vi "SDG60ConfArbWaveformOLD.vi"(0 "VISA resource name":refnum<visa-resource-name>="USB0::0xF4EC::0x1101::SDG6XEBC5R0119::INSTR", 1 "Freq/SR/P (1 Hz)":dbl=1000.0 min=1e-06 max=160000000.0 step=1.0 format="%#.15g", 2 "Phase (0.0 degrees)":dbl min=-360.0 max=360.0 format="%#.15g", 3 "Interpolation 0: Zero-order":i32(ring) items=["Zero-Order", "Linear", "Sinc", "Sin27", "Sinc13"], 5 "Select Channel (1:Channel 1)":i32(ring)=1 items=["Channel 1"=1, "Channel 2"=2], 7 "Amplitude (1.0 Vpp)":dbl=1.0 min=0.001 max=20.0 step=1.0 format="%#.15f", 9 "Select Freq/SR/P":i32(ring)=1 items=["Frequency", "Sample Rate", "Period"], 11 "error in (no error)":errorcluster, 12 "DC Offset (0.00 V)":dbl min=-10.0 max=10.0 format="%#_15g", 13 "DDS/TArb 0: DDS":i32(ring) items=["DDS", "TrueArb"]) -> (4 "VISA resource name out":refnum<visa-resource-name>, 15 "error out":errorcluster)   [LabVIEW 2018]
doc: "Sets the waveform parameters for an arbitrary waveform. This VI should be called after <b>Create Arbitrary Waveform.vi</b> (for user defined arbitrary waveform) and <b>Select Arbitrary Waveform.vi</b>"
panel:
  # "Sinc style interpolations use virtual keys\nVirtual keys not used for zero-hold & linear"
  # "2mVpp-20Vpp"
  # "For Period, TrueArb won't show on monitor-but will use (rounded value)\nFor SR, need to use TrueArb\nTo change interpolation method, use TrueArb\nMay take time to switch to TrueArb if WFM is large"
  # "Freq (DDS): 1uHz-50MHz \nFreq (TrueArb): 1uHz- Max depends on WFM length\nSR: 1uS/s-300MSa/s\nP: 20ns-1Ms\n10 Digit precision for F & SR\n6 Digit precision for P"
  # "TODO:  Choose Freq/period\namplitude/hi\noffset/low\nphase/delay"
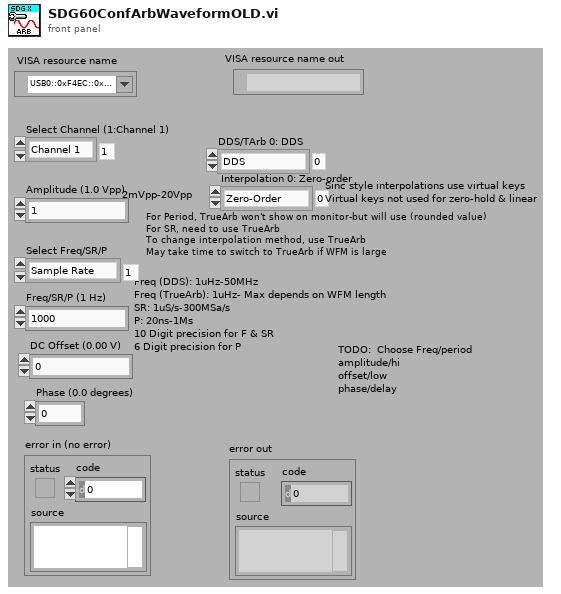
[diagram p1: front panel]
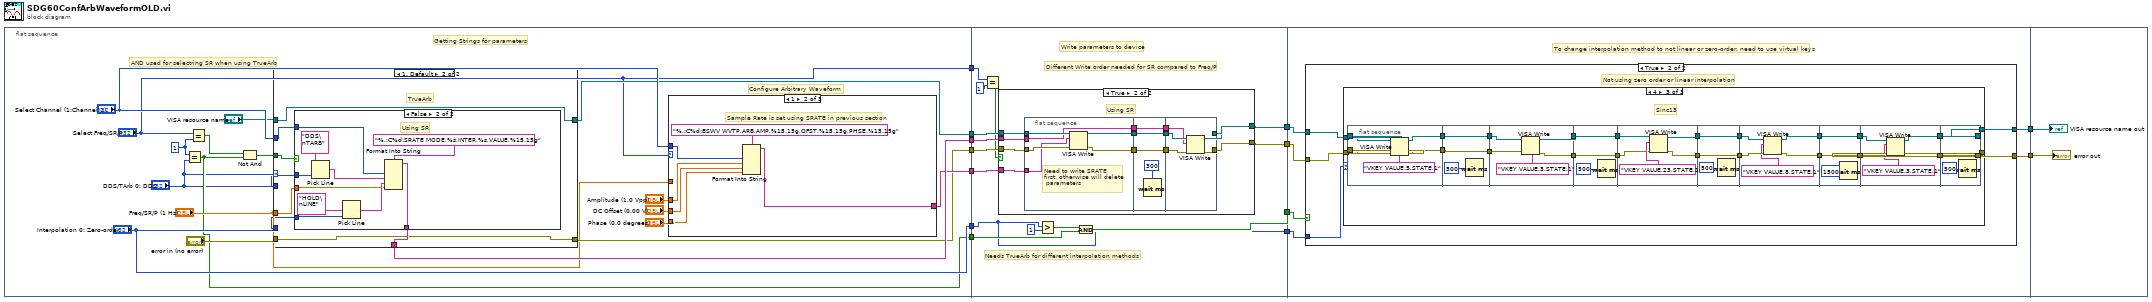
[diagram p0: block diagram]
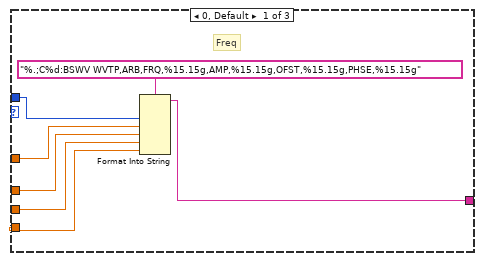
[diagram p2: hidden frame]
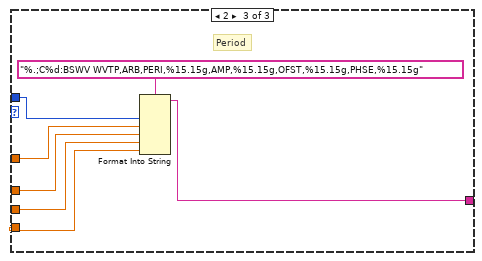
[diagram p3: hidden frame]
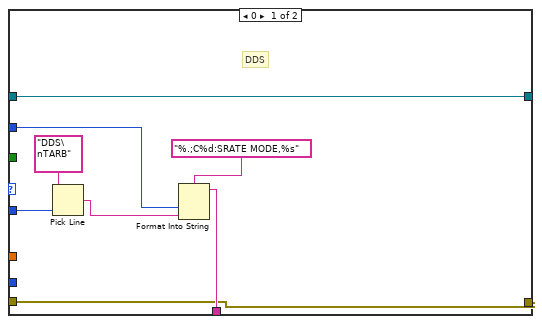
[diagram p4: hidden frame]
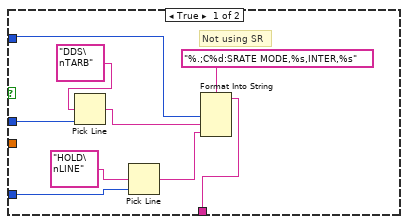
[diagram p5: hidden frame]
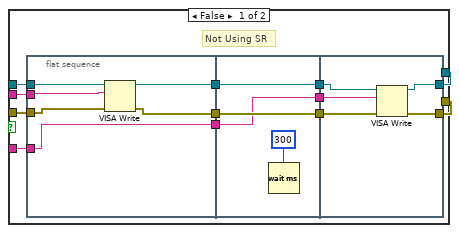
[diagram p6: hidden frame]
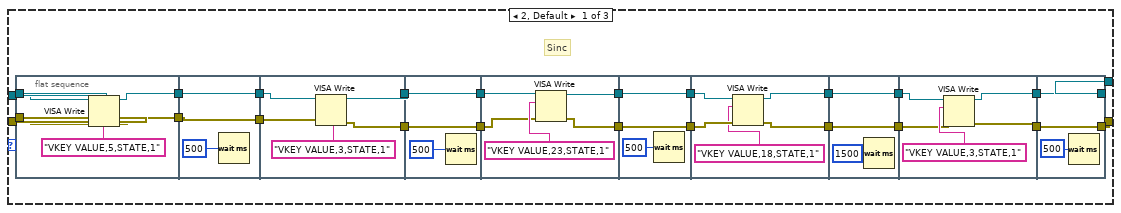
[diagram p8: hidden frame]
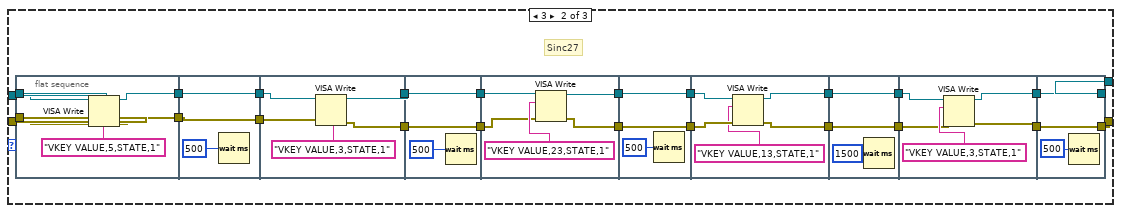
[diagram p9: hidden frame]
diagram:
  n1 = flat-sequence {
    tunnel: [w25] -> w13
    tunnel: [w24] -> w12
    tunnel: [w23] -> w11
    tunnel: [w22] -> w10
    tunnel: [w17] -> w9
    tunnel: ["Interpolation 0: Zero-order"] -> w8
    tunnel: ["Select Freq/SR/P"] -> w1
    tunnel: w13 -> [w100]
    tunnel: w12 -> [w99]
    tunnel: w11 -> [w98]
    tunnel: w10 -> [w97]
    tunnel: w9 -> [w93]
    tunnel: w8 -> [w90]
    tunnel: [w96] -> w7
    tunnel: [w95] -> w6
    tunnel: [w92] -> w5
    tunnel: [w90] -> w4
    tunnel: w1 -> [w88]
    tunnel: w7 -> [w159]
    tunnel: w6 -> [w158]
    tunnel: w5 -> [w160]
    tunnel: w4 -> [w157]
    tunnel: [w156] -> w3
    tunnel: [w155] -> w2
    tunnel: w3 -> [w354]
    tunnel: w2 -> [w355]
    frame #0 {
      w16 = 1
      # "Getting Strings for parameters"
      # "AND used for selectring SR when using TrueArb"
      # "Configure Arbitrary Waveform"
      n2 = Equal?(x=w16, y="DDS/TArb 0: DDS") -> (x = y?=w17:bool)
      n3 = Equal?(x="Select Freq/SR/P", y=w16) -> (x = y?=w18:bool)
      n4 = Not And(1:w17, 2:w18) -> (0:w15:bool)
      n5 = case shown="1, Default" "DDS/TArb 0: DDS" {
        tunnel: "Interpolation 0: Zero-order" -> [_ w67]
        tunnel: "DDS/TArb 0: DDS" -> [w58 w66]
        tunnel: "Select Channel (1:Channel 1)" -> [w56 w65]
        tunnel: [w55 w64] -> w25
        tunnel: w15 -> [_ w60]
        tunnel: "VISA resource name" -> [w53 w63]
        tunnel: "error in (no error)" -> [w52 w62]
        tunnel: [w53 w63] -> w22
        tunnel: [w52 w62] -> w23
        tunnel: "Freq/SR/P (1 Hz)" -> [_ w61]
        frame 0 {
          # "DDS"
          n6 = Pick Line(multi-line string="DDS\nTARB", line index=w58) -> (output string=w57:string)  [unwired: 1 in]
          n7 = Format Into String(format string="%.;C%d:SRATE MODE,%s", w56, w57) -> (resulting string=w55:string)  [unwired: 2 in, 1 out]
        }
        frame 1, Default {
          # "TrueArb"
          n8 = case shown="False" w60 {
            tunnel: w67 -> [w68 w85]
            tunnel: w66 -> [w70 w83]
            tunnel: w65 -> [w71 w81]
            tunnel: [w69 w80] -> w64
            tunnel: w61 -> [_ w77]
            frame True {
              # "Not using SR"
              n9 = Pick Line(multi-line string="DDS\nTARB", line index=w70) -> (output string=w76:string)  [unwired: 1 in]
              n10 = Pick Line(multi-line string="HOLD\nLINE", line index=w68) -> (output string=w75:string)  [unwired: 1 in]
              n11 = Format Into String(format string="%.;C%d:SRATE MODE,%s,INTER,%s", w71, w76, w75) -> (resulting string=w69:string)  [unwired: 2 in, 1 out]
            }
            frame False {
              # "Using SR"
              n12 = Pick Line(multi-line string="DDS\nTARB", line index=w83) -> (output string=w82:string)  [unwired: 1 in]
              n13 = Pick Line(multi-line string="HOLD\nLINE", line index=w85) -> (output string=w84:string)  [unwired: 1 in]
              n14 = Format Into String(format string="%.;C%d:SRATE MODE,%s,INTER,%s,VALUE,%15.15g", w81, w82, w84, w77) -> (resulting string=w80:string)  [unwired: 2 in, 1 out]
            }
          }
        }
      }
      n15 = case shown="1" "Select Freq/SR/P" {
        tunnel: "Freq/SR/P (1 Hz)" -> [w37 _ w50]
        tunnel: "Amplitude (1.0 Vpp)" -> [w36 w41 w49]
        tunnel: "DC Offset (0.00 V)" -> [w35 w40 w48]
        tunnel: "Phase (0.0 degrees)" -> [w34 w39 w47]
        tunnel: "Select Channel (1:Channel 1)" -> [w33 w43 w46]
        tunnel: [w32 w42 w45] -> w24
        frame 0, Default {
          # "Freq"
          n16 = Format Into String(format string="%.;C%d:BSWV WVTP,ARB,FRQ,%15.15g,AMP,%15.15g,OFST,%15.15g,PHSE,%15.15g", w33, w37, w36, w35, w34) -> (resulting string=w32:string)  [unwired: 2 in, 1 out]
        }
        frame 1 {
          # "Sample Rate is set using SRATE in previous section"
          n17 = Format Into String(format string="%.;C%d:BSWV WVTP,ARB,AMP,%15.15g,OFST,%15.15g,PHSE,%15.15g", w43, w41, w40, w39) -> (resulting string=w42:string)  [unwired: 2 in, 1 out]
        }
        frame 2 {
          # "Period"
          n18 = Format Into String(format string="%.;C%d:BSWV WVTP,ARB,PERI,%15.15g,AMP,%15.15g,OFST,%15.15g,PHSE,%15.15g", w46, w50, w49, w48, w47) -> (resulting string=w45:string)  [unwired: 2 in, 1 out]
        }
      }
    }
    frame #1 {
      # "Different Write order needed for SR compared to Freq/P"
      # "Write parameters to device"
      # "Needs TrueArb for different interpolation methods"
      n19 = Equal?(x=w88, y=1) -> (x = y?=w87:bool)
      n20 = case shown="True" w87 {
        tunnel: w100 -> [w106 w135]
        tunnel: w99 -> [w105 w134]
        tunnel: w98 -> [w104 w133]
        tunnel: w97 -> [w103 w132]
        tunnel: [w102 w131] -> w96
        tunnel: [w101 w130] -> w95
        frame False {
          # "Not Using SR"
          n21 = flat-sequence {
            tunnel: [w117] -> w112
            tunnel: w106 -> [w118]
            tunnel: [w116] -> w111
            tunnel: w105 -> [w115]
            tunnel: [w115] -> w110
            tunnel: w104 -> [w114]
            tunnel: w103 -> [w113]
            tunnel: w112 -> [w121]
            tunnel: [w121] -> w109
            tunnel: [w120] -> w108
            tunnel: w111 -> [w120]
            tunnel: w110 -> [w119]
            tunnel: [w119] -> w107
            tunnel: [w123] -> w102
            tunnel: w109 -> [w124]
            tunnel: w108 -> [w127]
            tunnel: [w126] -> w101
            tunnel: w107 -> [w125]
            frame #0 {
              n22 = VISA Write(VISA resource name=w113, write buffer=w118, error in (no error)=w114) -> (VISA resource name out=w117:refnum<visa-resource-name>, error out=w116:errorcluster)  [unwired: 1 out]
            }
            frame #1 {
              n23 = Wait (ms)(milliseconds to wait=300 ("x")) -> ()  [unwired: 1 out]
            }
            frame #2 {
              n24 = VISA Write(VISA resource name=w124, write buffer=w125, error in (no error)=w127) -> (VISA resource name out=w123:refnum<visa-resource-name>, error out=w126:errorcluster)  [unwired: 1 out]
            }
          }
        }
        frame True {
          # "Using SR"
          n25 = flat-sequence {
            tunnel: [w145] -> w139
            tunnel: w135 -> [w141]
            tunnel: [w144] -> w138
            tunnel: w134 -> [w140]
            tunnel: w133 -> [w143]
            tunnel: w132 -> [w142]
            tunnel: [w141] -> w128
            tunnel: w139 -> [w148]
            tunnel: [w148] -> w137
            tunnel: [w147] -> w136
            tunnel: w138 -> [w147]
            tunnel: [w146] -> w129
            tunnel: w128 -> [w146]
            tunnel: [w151] -> w131
            tunnel: w137 -> [w152]
            tunnel: w136 -> [w154]
            tunnel: [w153] -> w130
            tunnel: w129 -> [w150]
            frame #0 {
              # "Need to write SRATE\nfirst, otherwise will delete\n parameters"
              n26 = VISA Write(VISA resource name=w142, write buffer=w140, error in (no error)=w143) -> (VISA resource name out=w145:refnum<visa-resource-name>, error out=w144:errorcluster)  [unwired: 1 out]
            }
            frame #1 {
              n27 = Wait (ms)(milliseconds to wait=300 ("x")) -> ()  [unwired: 1 out]
            }
            frame #2 {
              n28 = VISA Write(VISA resource name=w152, write buffer=w150, error in (no error)=w154) -> (VISA resource name out=w151:refnum<visa-resource-name>, error out=w153:errorcluster)  [unwired: 1 out]
            }
          }
        }
      }
      n29 = Greater?(x=w90, y=1) -> (0:w94:bool)
      n30 = And(x=w94, y=w93) -> (x .and. y?=w92:bool)
    }
    frame #2 {
      # "To change interpolation method to not linear or zero-order, need to use virtual keys"
      n31 = case shown="True" w160 {
        tunnel: [w162 w163] -> w156
        tunnel: [w161 w164] -> w155
        tunnel: w159 -> [w162 w166]
        tunnel: w158 -> [w161 w165]
        tunnel: w157 -> [_ w167]
        frame False {
          # "Using Zero order or linear interpolation"
        }
        frame True {
          # "Not using zero order or linear interpolation"
          n32 = case shown="4" w167 {
            tunnel: w166 -> [w184 w246 w308]
            tunnel: w165 -> [w185 w247 w309]
            tunnel: [w182 w244 w306] -> w164
            tunnel: [w183 w245 w307] -> w163
            frame 2, Default {
              # "Sinc"
              n33 = flat-sequence {
                tunnel: w185 -> [w194]
                tunnel: w184 -> [w193]
                tunnel: [w192] -> w189
                tunnel: [w190] -> w188
                tunnel: w189 -> [w197]
                tunnel: [w197] -> w187
                tunnel: [w195] -> w186
                tunnel: w188 -> [w195]
                tunnel: w187 -> [w201]
                tunnel: w186 -> [w198]
                tunnel: [w200] -> w181
                tunnel: [w199] -> w180
                tunnel: w181 -> [w205]
                tunnel: [w205] -> w179
                tunnel: w180 -> [w204]
                tunnel: [w204] -> w177
                tunnel: w179 -> [w210]
                tunnel: [w206] -> w178
                tunnel: w177 -> [w208]
                tunnel: [w207] -> w176
                tunnel: w178 -> [w213]
                tunnel: w176 -> [w212]
                tunnel: [w213] -> w175
                tunnel: [w212] -> w174
                tunnel: w175 -> [w218]
                tunnel: w174 -> [w217]
                tunnel: [w215] -> w173
                tunnel: [w216] -> w172
                tunnel: w173 -> [w221]
                tunnel: w172 -> [w220]
                tunnel: [w221] -> w171
                tunnel: [w220] -> w170
                tunnel: w171 -> [w226]
                tunnel: w170 -> [w223]
                tunnel: [w225] -> w169
                tunnel: [w222] -> w168
                tunnel: [w228] -> w182
                tunnel: [w229] -> w183
                tunnel: w169 -> [w229]
                tunnel: w168 -> [w228]
                frame #0 {
                  n34 = VISA Write(VISA resource name=w193, write buffer="VKEY VALUE,5,STATE,1", error in (no error)=w194) -> (VISA resource name out=w192:refnum<visa-resource-name>, error out=w190:errorcluster)  [unwired: 1 out]
                }
                frame #1 {
                  n35 = Wait (ms)(milliseconds to wait=500) -> ()  [unwired: 1 out]
                }
                frame #2 {
                  n36 = VISA Write(VISA resource name=w201, write buffer="VKEY VALUE,3,STATE,1", error in (no error)=w198) -> (VISA resource name out=w200:refnum<visa-resource-name>, error out=w199:errorcluster)  [unwired: 1 out]
                }
                frame #3 {
                  n37 = Wait (ms)(milliseconds to wait=500) -> ()  [unwired: 1 out]
                }
                frame #4 {
                  n38 = VISA Write(VISA resource name=w210, write buffer="VKEY VALUE,23,STATE,1", error in (no error)=w208) -> (VISA resource name out=w206:refnum<visa-resource-name>, error out=w207:errorcluster)  [unwired: 1 out]
                }
                frame #5 {
                  n39 = Wait (ms)(milliseconds to wait=500) -> ()  [unwired: 1 out]
                }
                frame #6 {
                  n40 = VISA Write(VISA resource name=w218, write buffer="VKEY VALUE,18,STATE,1", error in (no error)=w217) -> (VISA resource name out=w215:refnum<visa-resource-name>, error out=w216:errorcluster)  [unwired: 1 out]
                }
                frame #7 {
                  n41 = Wait (ms)(milliseconds to wait=1500) -> ()  [unwired: 1 out]
                }
                frame #8 {
                  n42 = VISA Write(VISA resource name=w226, write buffer="VKEY VALUE,3,STATE,1", error in (no error)=w223) -> (VISA resource name out=w225:refnum<visa-resource-name>, error out=w222:errorcluster)  [unwired: 1 out]
                }
                frame #9 {
                  n43 = Wait (ms)(milliseconds to wait=500) -> ()  [unwired: 1 out]
                }
              }
            }
            frame 3 {
              # "Sinc27"
              n44 = flat-sequence {
                tunnel: w247 -> [w256]
                tunnel: w246 -> [w255]
                tunnel: [w254] -> w251
                tunnel: [w252] -> w250
                tunnel: w251 -> [w259]
                tunnel: [w259] -> w249
                tunnel: [w257] -> w248
                tunnel: w250 -> [w257]
                tunnel: w249 -> [w263]
                tunnel: w248 -> [w260]
                tunnel: [w262] -> w243
                tunnel: [w261] -> w242
                tunnel: w243 -> [w267]
                tunnel: [w267] -> w241
                tunnel: w242 -> [w266]
                tunnel: [w266] -> w239
                tunnel: w241 -> [w272]
                tunnel: [w268] -> w240
                tunnel: w239 -> [w270]
                tunnel: [w269] -> w238
                tunnel: w240 -> [w275]
                tunnel: w238 -> [w274]
                tunnel: [w275] -> w237
                tunnel: [w274] -> w236
                tunnel: w237 -> [w280]
                tunnel: w236 -> [w279]
                tunnel: [w277] -> w235
                tunnel: [w278] -> w234
                tunnel: w235 -> [w283]
                tunnel: w234 -> [w282]
                tunnel: [w283] -> w233
                tunnel: [w282] -> w232
                tunnel: w233 -> [w288]
                tunnel: w232 -> [w285]
                tunnel: [w287] -> w231
                tunnel: [w284] -> w230
                tunnel: [w290] -> w244
                tunnel: [w291] -> w245
                tunnel: w231 -> [w291]
                tunnel: w230 -> [w290]
                frame #0 {
                  n45 = VISA Write(VISA resource name=w255, write buffer="VKEY VALUE,5,STATE,1", error in (no error)=w256) -> (VISA resource name out=w254:refnum<visa-resource-name>, error out=w252:errorcluster)  [unwired: 1 out]
                }
                frame #1 {
                  n46 = Wait (ms)(milliseconds to wait=500) -> ()  [unwired: 1 out]
                }
                frame #2 {
                  n47 = VISA Write(VISA resource name=w263, write buffer="VKEY VALUE,3,STATE,1", error in (no error)=w260) -> (VISA resource name out=w262:refnum<visa-resource-name>, error out=w261:errorcluster)  [unwired: 1 out]
                }
                frame #3 {
                  n48 = Wait (ms)(milliseconds to wait=500) -> ()  [unwired: 1 out]
                }
                frame #4 {
                  n49 = VISA Write(VISA resource name=w272, write buffer="VKEY VALUE,23,STATE,1", error in (no error)=w270) -> (VISA resource name out=w268:refnum<visa-resource-name>, error out=w269:errorcluster)  [unwired: 1 out]
                }
                frame #5 {
                  n50 = Wait (ms)(milliseconds to wait=500) -> ()  [unwired: 1 out]
                }
                frame #6 {
                  n51 = VISA Write(VISA resource name=w280, write buffer="VKEY VALUE,13,STATE,1", error in (no error)=w279) -> (VISA resource name out=w277:refnum<visa-resource-name>, error out=w278:errorcluster)  [unwired: 1 out]
                }
                frame #7 {
                  n52 = Wait (ms)(milliseconds to wait=1500) -> ()  [unwired: 1 out]
                }
                frame #8 {
                  n53 = VISA Write(VISA resource name=w288, write buffer="VKEY VALUE,3,STATE,1", error in (no error)=w285) -> (VISA resource name out=w287:refnum<visa-resource-name>, error out=w284:errorcluster)  [unwired: 1 out]
                }
                frame #9 {
                  n54 = Wait (ms)(milliseconds to wait=500) -> ()  [unwired: 1 out]
                }
              }
            }
            frame 4 {
              # "Sinc13"
              n55 = flat-sequence {
                tunnel: w309 -> [w318]
                tunnel: w308 -> [w317]
                tunnel: [w316] -> w313
                tunnel: [w314] -> w312
                tunnel: w313 -> [w321]
                tunnel: [w321] -> w311
                tunnel: [w319] -> w310
                tunnel: w312 -> [w319]
                tunnel: w311 -> [w325]
                tunnel: w310 -> [w322]
                tunnel: [w324] -> w305
                tunnel: [w323] -> w304
                tunnel: w305 -> [w329]
                tunnel: [w329] -> w303
                tunnel: w304 -> [w328]
                tunnel: [w328] -> w301
                tunnel: w303 -> [w334]
                tunnel: [w330] -> w302
                tunnel: w301 -> [w332]
                tunnel: [w331] -> w300
                tunnel: w302 -> [w337]
                tunnel: w300 -> [w336]
                tunnel: [w337] -> w299
                tunnel: [w336] -> w298
                tunnel: w299 -> [w342]
                tunnel: w298 -> [w341]
                tunnel: [w339] -> w297
                tunnel: [w340] -> w296
                tunnel: w297 -> [w345]
                tunnel: w296 -> [w344]
                tunnel: [w345] -> w295
                tunnel: [w344] -> w294
                tunnel: w295 -> [w350]
                tunnel: w294 -> [w347]
                tunnel: [w349] -> w293
                tunnel: [w346] -> w292
                tunnel: [w352] -> w306
                tunnel: [w353] -> w307
                tunnel: w293 -> [w353]
                tunnel: w292 -> [w352]
                frame #0 {
                  n56 = VISA Write(VISA resource name=w317, write buffer="VKEY VALUE,5,STATE,1", error in (no error)=w318) -> (VISA resource name out=w316:refnum<visa-resource-name>, error out=w314:errorcluster)  [unwired: 1 out]
                }
                frame #1 {
                  n57 = Wait (ms)(milliseconds to wait=500) -> ()  [unwired: 1 out]
                }
                frame #2 {
                  n58 = VISA Write(VISA resource name=w325, write buffer="VKEY VALUE,3,STATE,1", error in (no error)=w322) -> (VISA resource name out=w324:refnum<visa-resource-name>, error out=w323:errorcluster)  [unwired: 1 out]
                }
                frame #3 {
                  n59 = Wait (ms)(milliseconds to wait=500) -> ()  [unwired: 1 out]
                }
                frame #4 {
                  n60 = VISA Write(VISA resource name=w334, write buffer="VKEY VALUE,23,STATE,1", error in (no error)=w332) -> (VISA resource name out=w330:refnum<visa-resource-name>, error out=w331:errorcluster)  [unwired: 1 out]
                }
                frame #5 {
                  n61 = Wait (ms)(milliseconds to wait=500) -> ()  [unwired: 1 out]
                }
                frame #6 {
                  n62 = VISA Write(VISA resource name=w342, write buffer="VKEY VALUE,8,STATE,1", error in (no error)=w341) -> (VISA resource name out=w339:refnum<visa-resource-name>, error out=w340:errorcluster)  [unwired: 1 out]
                }
                frame #7 {
                  n63 = Wait (ms)(milliseconds to wait=1500) -> ()  [unwired: 1 out]
                }
                frame #8 {
                  n64 = VISA Write(VISA resource name=w350, write buffer="VKEY VALUE,3,STATE,1", error in (no error)=w347) -> (VISA resource name out=w349:refnum<visa-resource-name>, error out=w346:errorcluster)  [unwired: 1 out]
                }
                frame #9 {
                  n65 = Wait (ms)(milliseconds to wait=500) -> ()  [unwired: 1 out]
                }
              }
            }
          }
        }
      }
    }
    frame #3 {
      "VISA resource name out" <- w354
      "error out" <- w355
    }
  }
